vi "Periodic Tasks.vi"(0 "error in":errorcluster) -> ()   [LabVIEW 2019]
doc: "All TeleOperated, Autonomous, and Test controller logic are located here. Sensor reads and actuator commands are run inside of parallel loops. Most FRC 4265 code should be placed here."
uses:
  dsdata.vi
  dsinstructions.vi
  constants.vi
  outputs.vi
  autoninfo.vi
  sensors.vi
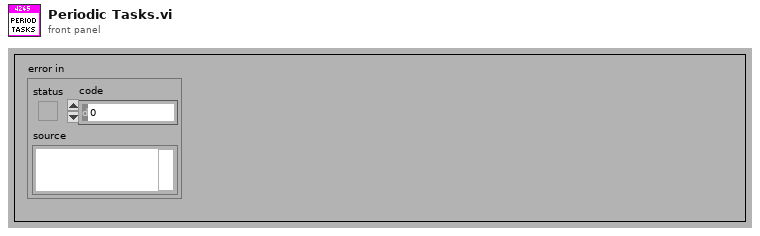
[diagram p1: front panel]
types:
  T1 = typedef "WPI_DriverStationRobotMode2.ctl" = enum16{"Autonomous Disabled", "Autonomous Enabled", "Teleop Disabled", "Teleop Enabled", "Disconnected", "Finish", "Test Disabled", "Test Enabled", "Emergency Stopped"}
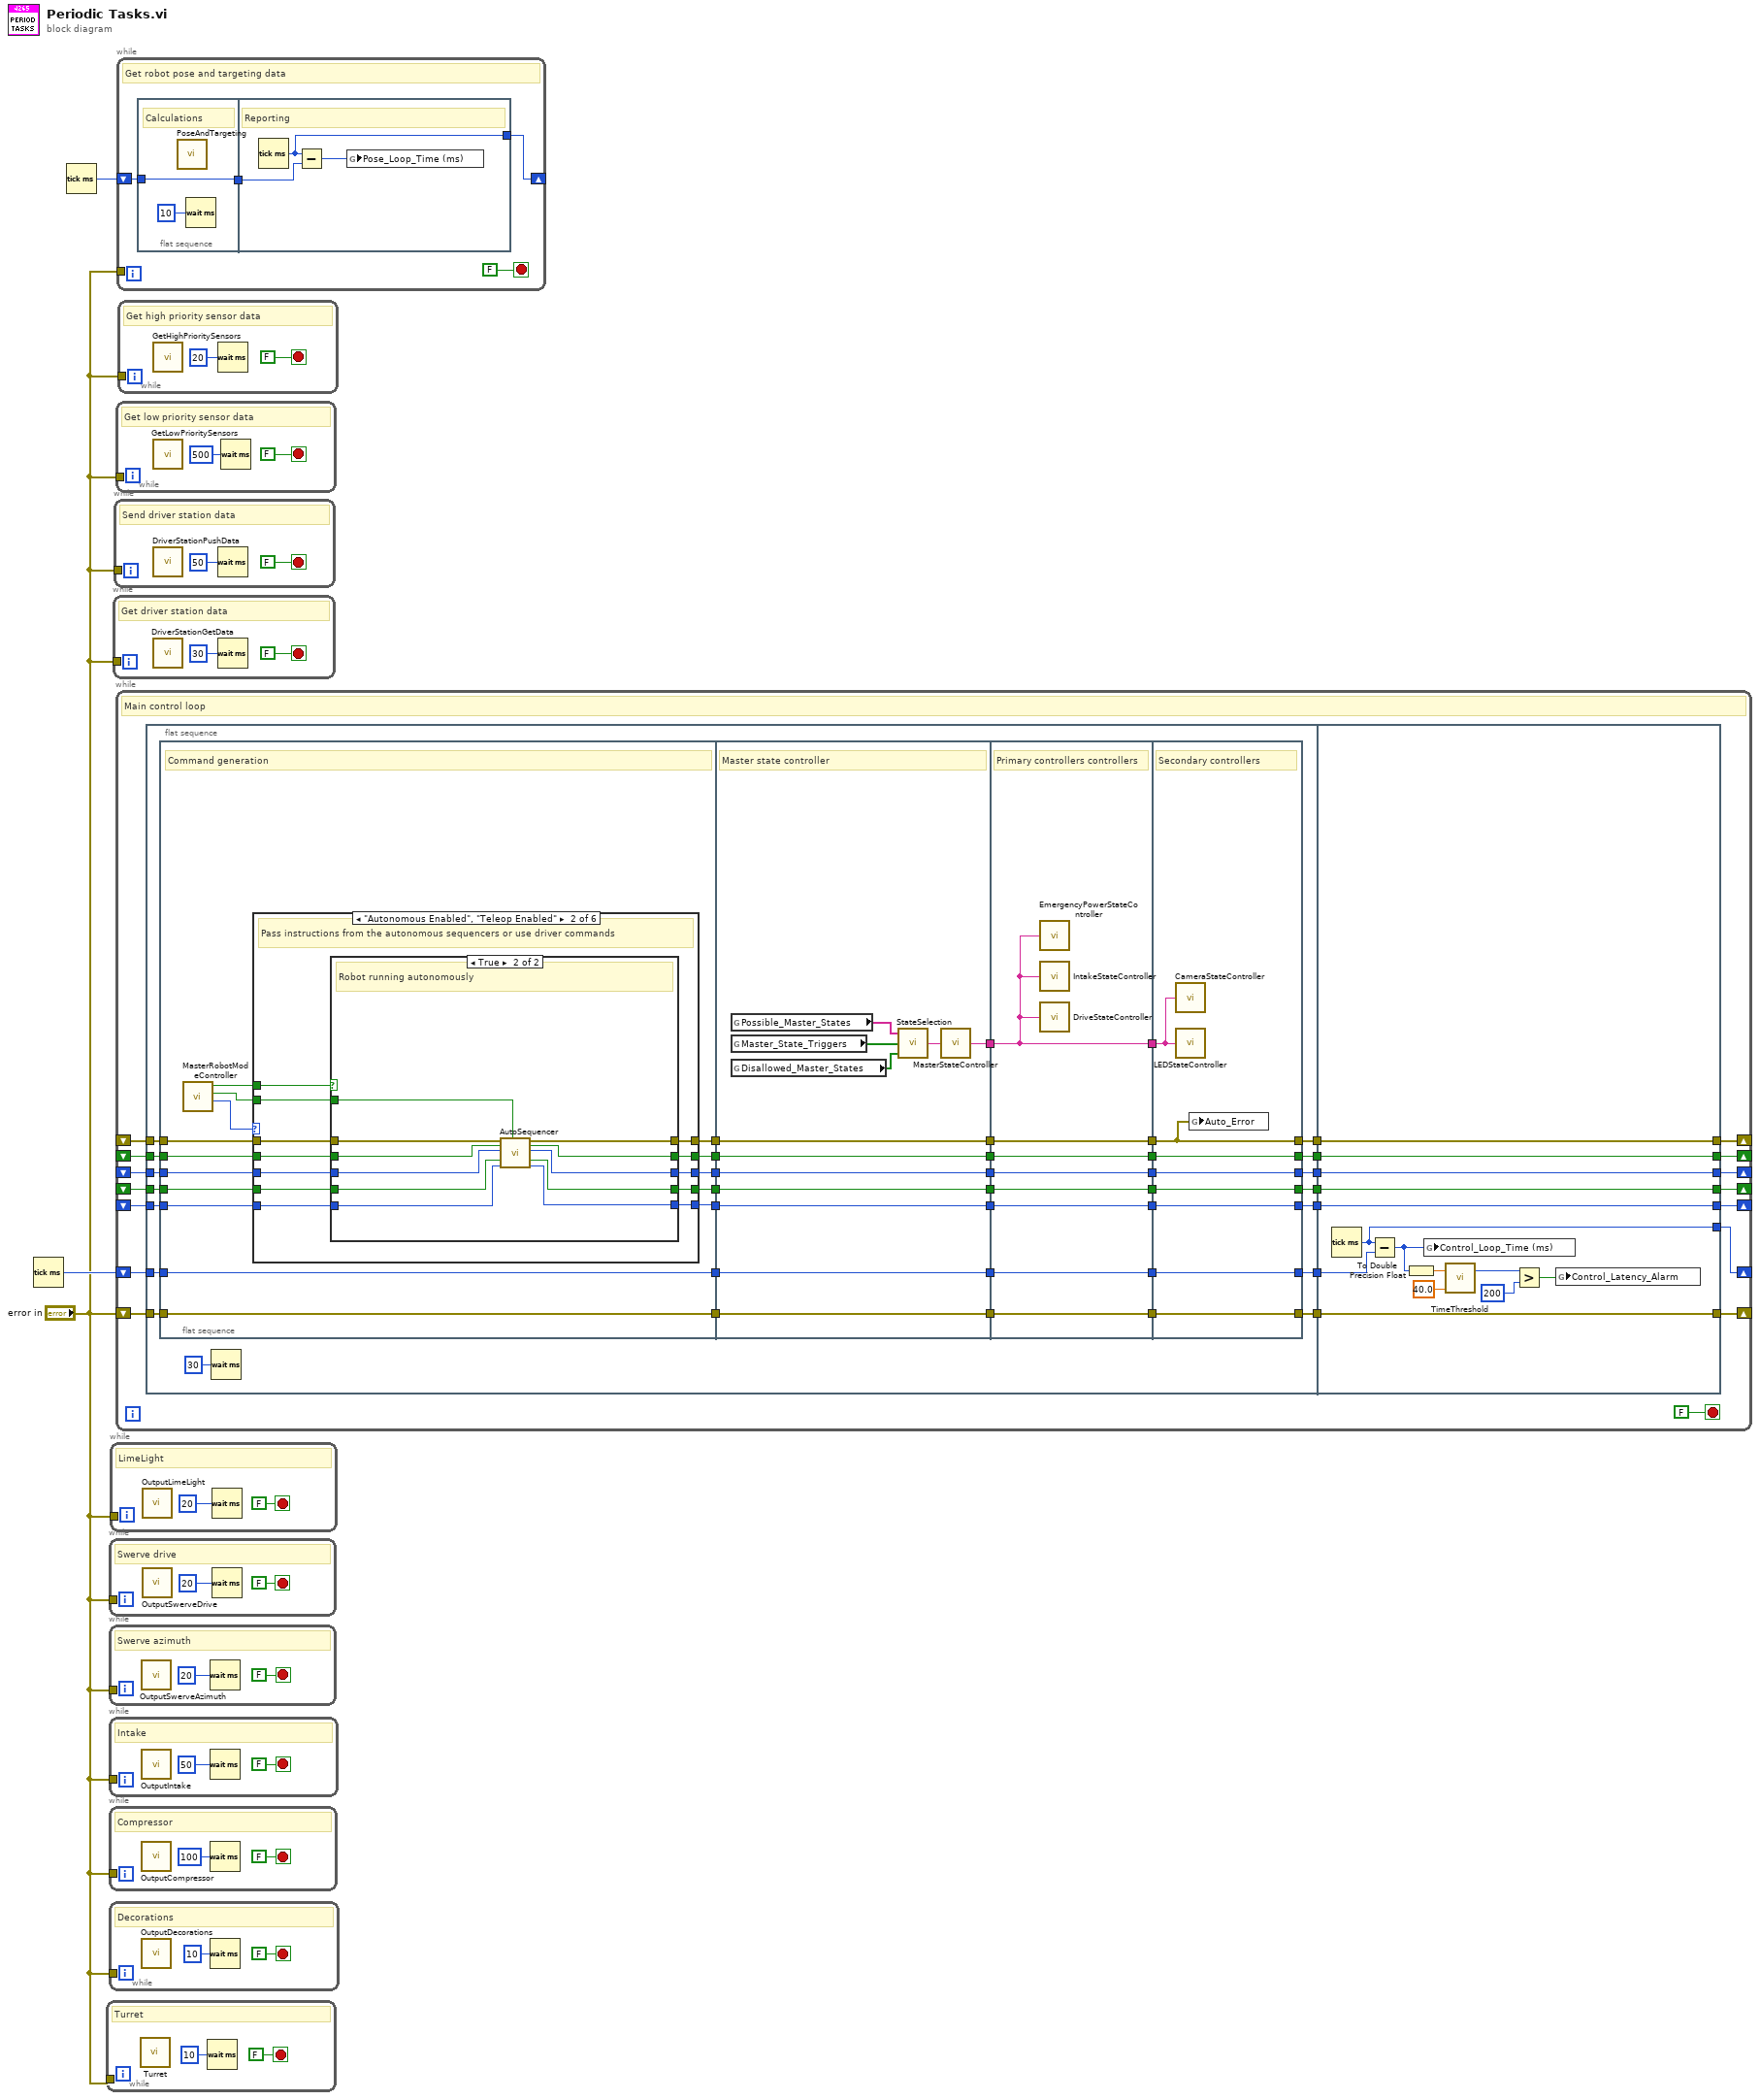
[diagram p0: block diagram]
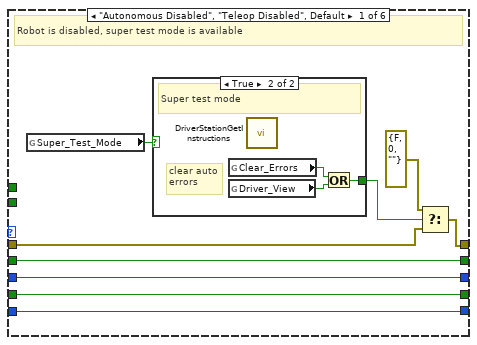
[diagram p2: hidden frame]
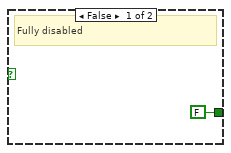
[diagram p3: hidden frame]
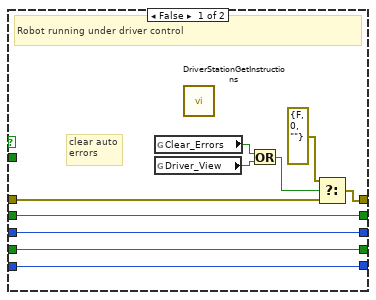
[diagram p4: hidden frame]
diagram:
  n1 = Tick Count (ms)() -> (millisecond timer value=w3:u32)
  n2 = Tick Count (ms)() -> (millisecond timer value=w2:u32)
  n3 = while {
    tunnel: "error in" -> [_]
    stop <- FALSE stop-if-true
    # "Turret"
    n4 = call "Turret.vi"() -> ()  [unwired: 12 in]
    n5 = Wait (ms)(milliseconds to wait=u32 10) -> ()  [unwired: 1 out]
  }
  n6 = while {
    tunnel: "error in" -> [_]
    stop <- FALSE stop-if-true
    # "Swerve drive"
    n7 = call "OutputSwerveDrive.vi"() -> ()  [unwired: 1 in]
    n8 = Wait (ms)(milliseconds to wait=u32 20) -> ()  [unwired: 1 out]
  }
  n9 = while {
    tunnel: "error in" -> [_]
    stop <- FALSE stop-if-true
    # "Swerve azimuth"
    n10 = call "OutputSwerveAzimuth.vi"() -> ()  [unwired: 1 in]
    n11 = Wait (ms)(milliseconds to wait=u32 20) -> ()  [unwired: 1 out]
  }
  n12 = while {
    tunnel: "error in" -> [_]
    stop <- FALSE stop-if-true
    # "Intake"
    n13 = call "OutputIntake.vi"() -> ()  [unwired: 1 in]
    n14 = Wait (ms)(milliseconds to wait=u32 50) -> ()  [unwired: 1 out]
  }
  n15 = while {
    tunnel: "error in" -> [_]
    stop <- FALSE stop-if-true
    # "Compressor"
    n16 = call "OutputCompressor.vi"() -> ()  [unwired: 1 in]
    n17 = Wait (ms)(milliseconds to wait=u32 100) -> ()  [unwired: 1 out]
  }
  n18 = while {
    tunnel: "error in" -> [_]
    stop <- FALSE stop-if-true
    # "Decorations"
    n19 = call "OutputDecorations.vi"() -> ()  [unwired: 1 in]
    n20 = Wait (ms)(milliseconds to wait=u32 10) -> ()  [unwired: 1 out]
  }
  n21 = while {
    tunnel: "error in" -> [_]
    stop <- FALSE stop-if-true
    # "LimeLight"
    n22 = call "OutputLimeLight.vi"() -> ()  [unwired: 1 in]
    n23 = Wait (ms)(milliseconds to wait=u32 20) -> ()  [unwired: 1 out]
  }
  n24 = while {
    tunnel: "error in" -> [_]
    stop <- FALSE stop-if-true
    # "Get driver station data"
    n25 = call "DriverStationGetData.vi"() -> ()  [unwired: 1 in]
    n26 = Wait (ms)(milliseconds to wait=u32 30) -> ()  [unwired: 1 out]
  }
  n27 = while {
    tunnel: "error in" -> [_]
    stop <- FALSE stop-if-true
    # "Send driver station data"
    n28 = call "DriverStationPushData.vi"() -> ()  [unwired: 12 in]
    n29 = Wait (ms)(milliseconds to wait=u32 50) -> ()  [unwired: 1 out]
  }
  n30 = while {
    tunnel: "error in" -> [_]
    stop <- FALSE stop-if-true
    # "Get low priority sensor data"
    n31 = call "GetLowPrioritySensors.vi"() -> ()  [unwired: 12 in]
    n32 = Wait (ms)(milliseconds to wait=u32 500) -> ()  [unwired: 1 out]
  }
  n33 = while {
    shift-right: [w41] -> _
    shift-left: _ -> [w43]
    shift-right: [w42] -> _
    shift-left: _ -> [w44]
    shift-right: [w40] -> _
    shift-left: _ -> [w39]
    shift-right: [w38] -> _
    shift-left: _ -> [w37]
    shift-right: [w31] -> _
    shift-left: w3 -> [w32]
    shift-right: [w36] -> _
    shift-left: _ -> [w35]
    shift-right: [w33] -> _
    shift-left: "error in" -> [w34]
    stop <- FALSE stop-if-true
    # "Main control loop"
    n34 = flat-sequence {
      tunnel: w44 -> [w61]
      tunnel: w43 -> [w60]
      tunnel: w39 -> [w56]
      tunnel: w37 -> [w54]
      tunnel: w35 -> [w52]
      tunnel: w34 -> [w51]
      tunnel: w32 -> [w49]
      tunnel: [w59] -> w30
      tunnel: [w58] -> w29
      tunnel: [w57] -> w28
      tunnel: [w55] -> w27
      tunnel: [w53] -> w26
      tunnel: [w50] -> w25
      tunnel: [w47] -> w24
      tunnel: [w193] -> w31
      tunnel: [w201] -> w33
      tunnel: [w202] -> w36
      tunnel: [w203] -> w38
      tunnel: [w204] -> w40
      tunnel: [w205] -> w41
      tunnel: [w206] -> w42
      tunnel: w30 -> [w206]
      tunnel: w29 -> [w205]
      tunnel: w28 -> [w204]
      tunnel: w27 -> [w203]
      tunnel: w26 -> [w202]
      tunnel: w25 -> [w201]
      tunnel: w24 -> [w194]
      frame #0 {
        n35 = flat-sequence {
          tunnel: w61 -> [w96]
          tunnel: w60 -> [w95]
          tunnel: [w98] -> w83
          tunnel: [w97] -> w82
          tunnel: [w94] -> w81
          tunnel: w56 -> [w93]
          tunnel: [w92] -> w80
          tunnel: w54 -> [w91]
          tunnel: [w90] -> w79
          tunnel: w52 -> [w89]
          tunnel: [w85] -> w78
          tunnel: w51 -> [w85]
          tunnel: [w84] -> w77
          tunnel: w49 -> [w84]
          tunnel: w83 -> [w165]
          tunnel: w82 -> [w176]
          tunnel: w81 -> [w175]
          tunnel: w80 -> [w174]
          tunnel: [w165] -> w76
          tunnel: [w176] -> w75
          tunnel: [w175] -> w74
          tunnel: [w174] -> w73
          tunnel: [w170] -> w72
          tunnel: [w169] -> w71
          tunnel: w79 -> [w169]
          tunnel: w78 -> [w168]
          tunnel: [w168] -> w70
          tunnel: w77 -> [w166]
          tunnel: [w166] -> w69
          tunnel: w76 -> [w184]
          tunnel: w75 -> [w183]
          tunnel: w74 -> [w182]
          tunnel: w73 -> [w181]
          tunnel: w72 -> [w177]
          tunnel: [w184] -> w68
          tunnel: [w183] -> w67
          tunnel: [w182] -> w66
          tunnel: [w181] -> w65
          tunnel: [w180] -> w64
          tunnel: w71 -> [w180]
          tunnel: [w179] -> w63
          tunnel: w70 -> [w179]
          tunnel: [w178] -> w62
          tunnel: w69 -> [w178]
          tunnel: [w177] -> w46
          tunnel: [w189] -> w55
          tunnel: [w190] -> w57
          tunnel: [w191] -> w58
          tunnel: [w192] -> w59
          tunnel: w68 -> [w192]
          tunnel: w67 -> [w191]
          tunnel: w66 -> [w190]
          tunnel: w65 -> [w189]
          tunnel: [w188] -> w53
          tunnel: w64 -> [w188]
          tunnel: [w187] -> w50
          tunnel: w63 -> [w187]
          tunnel: w62 -> [w186]
          tunnel: [w186] -> w47
          tunnel: w46 -> [w185]
          frame #0 {
            # "Command generation"
            n36 = call "MasterRobotModeController.vi"() -> ("FMS Robot Mode"=w88:T1, "Auto Reset"=w87:bool, "Robot is Autonomous"=w86:bool)  [unwired: 5 in]
            n37 = case shown="\"Autonomous Enabled\", \"Teleop Enabled\"" w88 {
              tunnel: w96 -> [w107 w120 w147 w152 w157 w162]
              tunnel: w95 -> [w106 w121 w146 w151 w156 w161]
              tunnel: [w107 w122 w147 w152 w157 w162] -> w98
              tunnel: [w106 w123 w146 w151 w156 w161] -> w97
              tunnel: w87 -> [_ w113 _ _ _ _]
              tunnel: [w105 w117 w148 w153 w158 w163] -> w94
              tunnel: w93 -> [w105 w115 w148 w153 w158 w163]
              tunnel: [w104 w116 w149 w154 w159 w164] -> w92
              tunnel: w91 -> [w104 w114 w149 w154 w159 w164]
              tunnel: [w101 w119 w145 w150 w155 w160] -> w90
              tunnel: w89 -> [w102 w118 w145 w150 w155 w160]
              tunnel: w86 -> [_ w112 _ _ _ _]
              frame "Autonomous Disabled", "Teleop Disabled", Default {
                # "Robot is disabled, super test mode is available"
                n38 = global read "dsdata.vi" "Super_Test_Mode"() -> (w103:bool)
                n39 = case shown="True" w103 {
                  tunnel: [FALSE w109] -> w99
                  frame False {
                    # "Fully disabled"
                  }
                  frame True {
                    # "clear auto\nerrors"
                    # "Super test mode"
                    n40 = global read "dsdata.vi" "Clear_Errors"() -> (w110:bool)
                    n41 = global read "dsinstructions.vi" "Driver_View"() -> (w111:bool)
                    n42 = call "DriverStationGetInstructions.vi"() -> ()  [unwired: 12 in]
                    n43 = Or(x=w110, y=w111) -> (x .or. y?=w109:bool)
                  }
                }
                n44 = Select(t=errorcluster {"status"=FALSE, "code"=0, "source"=""} ("Auto Error Out"), s=w99, f=w102) -> (s? t:f=w101:errorcluster)
              }
              frame "Autonomous Enabled", "Teleop Enabled" {
                # "Pass instructions from the autonomous sequencers or use driver commands"
                n45 = case shown="True" w112 {
                  tunnel: w113 -> [_ w136]
                  tunnel: [w124 w144] -> w123
                  tunnel: [w125 w143] -> w122
                  tunnel: w121 -> [w124 w142]
                  tunnel: w120 -> [w125 w141]
                  tunnel: [w128 w135] -> w119
                  tunnel: w118 -> [w129 w134]
                  tunnel: [w126 w140] -> w117
                  tunnel: [w127 w139] -> w116
                  tunnel: w115 -> [w126 w138]
                  tunnel: w114 -> [w127 w137]
                  frame False {
                    # "clear auto\nerrors"
                    # "Robot running under driver control"
                    n46 = global read "dsdata.vi" "Clear_Errors"() -> (w131:bool)
                    n47 = global read "dsinstructions.vi" "Driver_View"() -> (w132:bool)
                    n48 = call "DriverStationGetInstructions.vi"() -> ()  [unwired: 12 in]
                    n49 = Or(x=w131, y=w132) -> (x .or. y?=w133:bool)
                    n50 = Select(t=errorcluster {"status"=FALSE, "code"=0, "source"=""} ("Auto Error Out"), s=w133, f=w129) -> (s? t:f=w128:errorcluster)
                  }
                  frame True {
                    # "Robot running autonomously"
                    n51 = call "AutoSequencer.vi"("Auto Error In"=w134, "Mobility Advance In"=w137, "Mobility Step In"=w138, "Subsystem Advance In"=w141, "Subsystem Step In"=w142, "Reinit Sequencer"=w136) -> ("Auto Error Out"=w135:errorcluster, "Mobility Advance Out"=w139:bool, "Mobility Step Out"=w140:i32, "Subsystem Advance Out"=w143:bool, "Subsystem Step Out"=w144:i32)  [unwired: 9 in]
                  }
                }
              }
              frame "Finish" {
                # "Clean up operations are in the Finish.vi in RobotMain.vi"
              }
              frame "Test Disabled", "Test Enabled" {
                # "Use TestActuatorInterlock.vi for implimenting test code"
              }
              frame "Disconnected" {
                # "Communications have failed"
              }
              frame "Emergency Stopped" {
                # "Robot has been emergency stopped"
              }
            }
          }
          frame #1 {
            # "Master state controller"
            n52 = global read "constants.vi" "Possible_Master_States"() -> (w172:string[])
            n53 = global read "dsinstructions.vi" "Master_State_Triggers"() -> (w173:bool[])
            n54 = global read "outputs.vi" "Disallowed_Master_States"() -> (w167:bool[])
            n55 = call "StateSelection.vi"("Disallowed States"=w167, "State Triggers"=w173, "State Names"=w172) -> ("Selected State"=w171:string)
            n56 = call "MasterStateController.vi"("Selected State"=w171) -> ("Master State"=w170:string)
          }
          frame #2 {
            # "Primary controllers controllers"
            n57 = call "EmergencyPowerStateController.vi"("Master State"=w177) -> ()  [unwired: 1 in]
            n58 = call "IntakeStateController.vi"("Selected State (In)"=w177) -> ()  [unwired: 1 in]
            n59 = call "DriveStateController.vi"("Master State"=w177) -> ()  [unwired: 1 in]
          }
          frame #3 {
            # "Secondary controllers"
            n60 = call "CameraStateController.vi"("Master State"=w185) -> ()  [unwired: 1 in]
            n61 = call "LEDStateController.vi"("Master State"=w185) -> ()  [unwired: 1 in]
            n62 = global write "autoninfo.vi" "Auto_Error"(w188) -> ()
          }
        }
        n63 = Wait (ms)(milliseconds to wait=u32 30) -> ()  [unwired: 1 out]
      }
      frame #1 {
        n64 = Tick Count (ms)() -> (millisecond timer value=w193:u32)
        n65 = Subtract(x=w193, y=w194) -> (x-y=w200:u32)
        n66 = To Double Precision Float(number=w200) -> (double precision float=w199:dbl)
        n67 = global write "sensors.vi" "Control_Loop_Time (ms)"(w200) -> ()
        n68 = call "TimeThreshold.vi"("Threshold"=40.0, "Current Value"=w199) -> ("Time Above Threshold (ms)"=w198:u32)  [unwired: 1 out]
        n69 = Greater?(x=w198, y=u32 200) -> (0:w197:bool)
        n70 = global write "sensors.vi" "Control_Latency_Alarm"(w197) -> ()
      }
    }
  }
  n71 = while {
    tunnel: "error in" -> [_]
    shift-right: [w209] -> _
    shift-left: w2 -> [w208]
    stop <- FALSE stop-if-true
    # "Get robot pose and targeting data"
    n72 = flat-sequence {
      tunnel: w208 -> [w212]
      tunnel: [w212] -> w207
      tunnel: [w214] -> w209
      tunnel: w207 -> [w213]
      frame #0 {
        # "Calculations"
        n73 = call "PoseAndTargeting.vi"() -> ()  [unwired: 1 in]
        n74 = Wait (ms)(milliseconds to wait=u32 10) -> ()  [unwired: 1 out]
      }
      frame #1 {
        # "Reporting"
        n75 = Tick Count (ms)() -> (millisecond timer value=w214:u32)
        n76 = Subtract(x=w214, y=w213) -> (x-y=w215:u32)
        n77 = global write "sensors.vi" "Pose_Loop_Time (ms)"(w215) -> ()
      }
    }
  }
  n78 = while {
    tunnel: "error in" -> [_]
    stop <- FALSE stop-if-true
    # "Get high priority sensor data"
    n79 = call "GetHighPrioritySensors.vi"() -> ()  [unwired: 1 in]
    n80 = Wait (ms)(milliseconds to wait=u32 20) -> ()  [unwired: 1 out]
  }
